vi "2182Delta_LV71.vi"() -> ()   [LabVIEW 2019]
panel:
  in  "stop":bool
  out "Resistance of DUT":dbl[](graph)
  out "Resistance (mOhms)":dbl[](array[numeric]) format="%.10f"
  out "Voltage Drop Across DUT":dbl[](graph)
  out "Delta Readings (uV)":dbl[](array[numeric]) format="%.12f"
  in  "2400 CURR":dbl
  in  "2400 GPIB add":string="24"
  in  "2182 GPIB add":string="25"
  # "Ultra Low Resistance - Delta Mode Measurements using 2400 and 2182."
  # "KEITHLEY"
  # "Connect Trigger Link Cable between 2182 & 2400.\nNote that moving average (digital) filter is on by default,\navg = 10rdgs, window = 0.01%"
  # "Note: If you change 2182 Buffer points you must also change 2400 Trigger count to \n2 x 2182 buffer points. You should also set the Sample count to display = 2182 Buffer Points.\nAlso change R=V/I calculation if you use different current!"
  # "Note: Change R=V/I in the program, if you change current!"
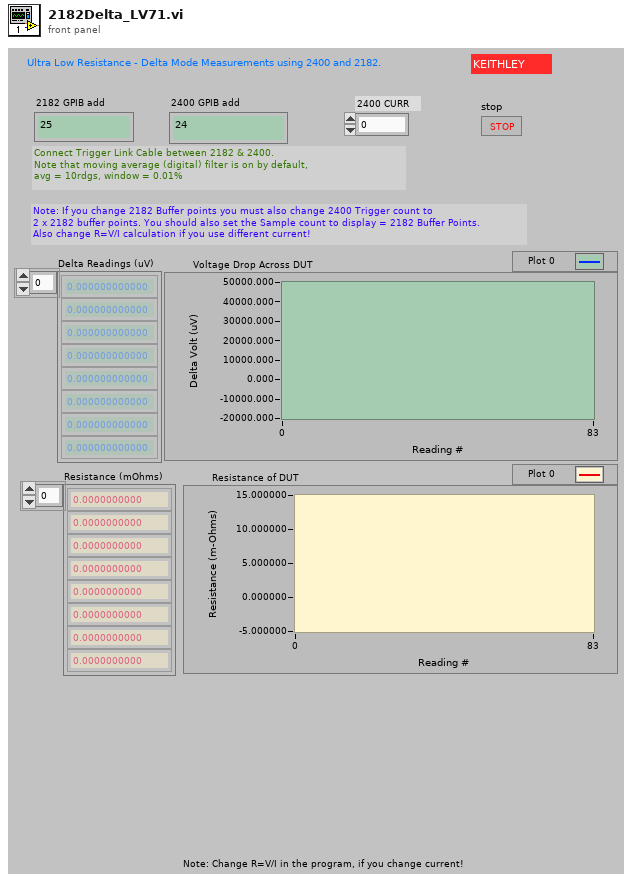
[diagram p1: front panel]
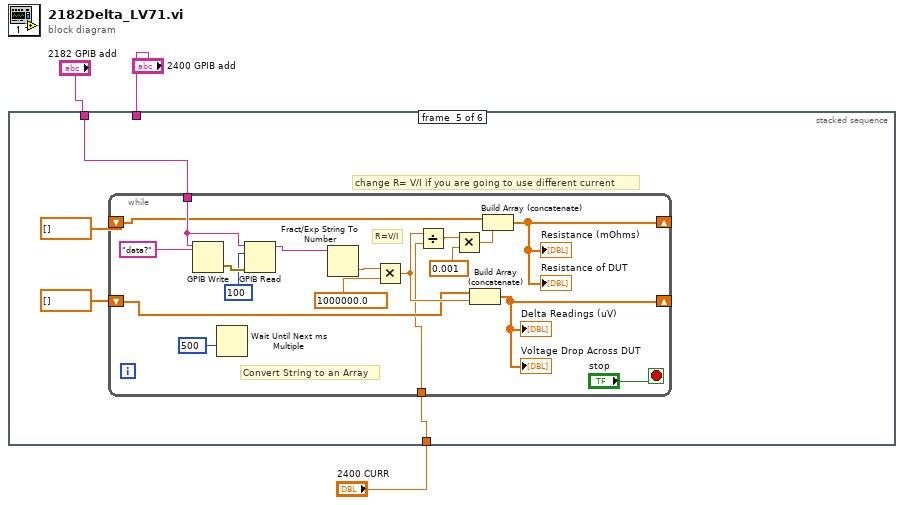
[diagram p0: block diagram]
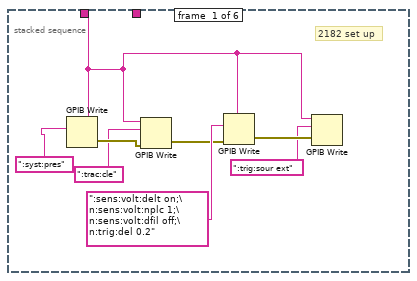
[diagram p2: hidden frame]
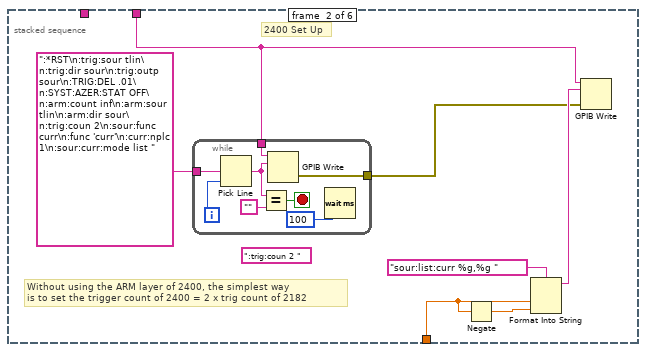
[diagram p3: hidden frame]
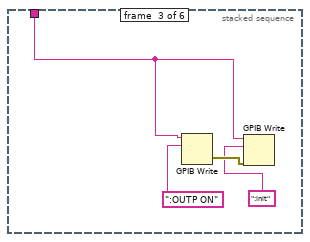
[diagram p4: hidden frame]
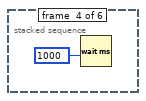
[diagram p5: hidden frame]
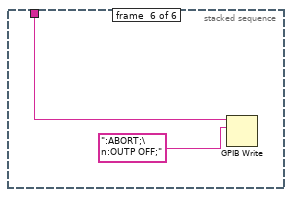
[diagram p6: hidden frame]
diagram:
  n1 = stacked-sequence {
    tunnel: "2182 GPIB add" -> [w5 _ _ _ w35 _]
    tunnel: "2400 GPIB add" -> [_ w12 w27 _ _ w55]
    tunnel: "2400 CURR" -> [_ w15 _ _ w34 _]
    frame #0 {
      # "2182 set up"
      n2 = GPIB Write(0:w5, 1:":syst:pres") -> (6:w11:errorcluster)  [unwired: 3 in, 1 out]
      n3 = GPIB Write(0:w5, 1:":trac:cle", 3:w11) -> (6:w4:errorcluster)  [unwired: 2 in, 1 out]
      n4 = GPIB Write(0:w5, 1:":sens:volt:delt on;\n:sens:volt:nplc 1;\n:sens:volt:dfil off;\n:trig:del 0.2", 3:w4) -> (6:w8:errorcluster)  [unwired: 2 in, 1 out]
      n5 = GPIB Write(0:w5, 1:":trig:sour ext", 3:w8) -> ()  [unwired: 2 in, 2 out]
    }
    frame #1 {
      (unwired) ":trig:coun 2 "
      # "Without using the ARM layer of 2400, the simplest way\nis to set the trigger count of 2400 = 2 x trig count of 2182"
      # "2400 Set Up"
      n6 = while {
        tunnel: ":*RST\n:trig:sour tlin\n:trig:dir sour\n:trig:outp sour\n:TRIG:DEL .01\n:SYST:AZER:STAT OFF\n:arm:count inf\n:arm:sour tlin\n:arm:dir sour\n:trig:coun 2\n:sour:func curr\n:func 'curr'\n:curr:nplc 1\n:sour:curr:mode list " -> [w25]
        tunnel: [w21] -> w13
        tunnel: w12 -> [w20]
        i -> [w26]
        stop <- w24 stop-if-true
        n7 = Pick Line(multi-line string=w25, line index=w26) -> (output string=w22:string)  [unwired: 1 in]
        n8 = Equal?(x=w22, y="") -> (x = y?=w24:bool)
        n9 = GPIB Write(0:w20, 1:w22) -> (6:w21:errorcluster)  [unwired: 3 in, 1 out]
        n10 = Wait (ms)(milliseconds to wait=u32 100) -> ()  [unwired: 1 out]
      }
      n11 = Negate(x=w15) -> (-x=w18:dbl)
      n12 = Format Into String(format string="sour:list:curr %g,%g ", w15, w18) -> (resulting string=w17:string)  [unwired: 2 in, 1 out]
      n13 = GPIB Write(0:w12, 1:w17, 3:w13) -> ()  [unwired: 2 in, 2 out]
    }
    frame #2 {
      n14 = GPIB Write(0:w27, 1:":OUTP ON") -> (6:w30:errorcluster)  [unwired: 3 in, 1 out]
      n15 = GPIB Write(0:w27, 1:":init", 3:w30) -> ()  [unwired: 2 in, 2 out]
    }
    frame #3 {
      n16 = Wait (ms)(milliseconds to wait=u32 1000) -> ()  [unwired: 1 out]
    }
    frame #4 {
      # "change R= V/I if you are going to use different current"
      n17 = while {
        tunnel: w35 -> [w48]
        tunnel: w34 -> [w43]
        shift-right: [w39] -> _
        shift-left: dbl[] [] -> [w44]
        shift-right: [w38] -> _
        shift-left: dbl[] [] -> [w45]
        stop <- "stop" stop-if-true
        # "R=V/I"
        # "Convert String to an Array"
        n18 = GPIB Write(0:w48, 1:"data?" ("data")) -> (6:w49:errorcluster)  [unwired: 3 in, 1 out]
        n19 = Wait Until Next ms Multiple(millisecond multiple=u32 500) -> ()  [unwired: 1 out]
        n20 = GPIB Read(0:w48, 1:100 ("byte count"), 3:w49) -> (5:w46:string)  [unwired: 2 in, 2 out]
        n21 = Fract/Exp String To Number(string=w46) -> (number=w50:dbl)  [unwired: 3 in, 1 out]
        n22 = Multiply(x=w50, y=1000000.0) -> (x*y=w51:dbl)
        n23 = Divide(x=w51, y=w43) -> (x/y=w52:dbl)
        n24 = Multiply(x=w52, y=0.001) -> (x*y=w42:dbl)
        n25 = Build Array (concatenate)(w44, w51) -> (w39:dbl[])
        "Delta Readings (uV)" <- w39
        "Voltage Drop Across DUT" <- w39
        n26 = Build Array (concatenate)(w45, w42) -> (w38:dbl[])
        "Resistance (mOhms)" <- w38
        "Resistance of DUT" <- w38
      }
    }
    frame #5 {
      n27 = GPIB Write(0:w55, 1:":ABORT;\n:OUTP OFF;" ("data")) -> ()  [unwired: 3 in, 2 out]
    }
  }
